vi "Read Children Tag.vi"(9 "Tag In":string, 11 "Tree in":refnum<class "Tree.lvclass">) -> (1 "Children Tag Out":string[](array[string]), 3 "Tree out":refnum<class "Tree.lvclass">)   [LabVIEW 2019, in "Tree.lvclass"]
uses:
  Tree.lvclass
  Tree.lvclass/Tree.ctl
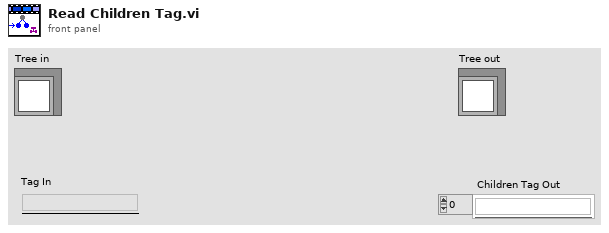
[diagram p1: front panel]
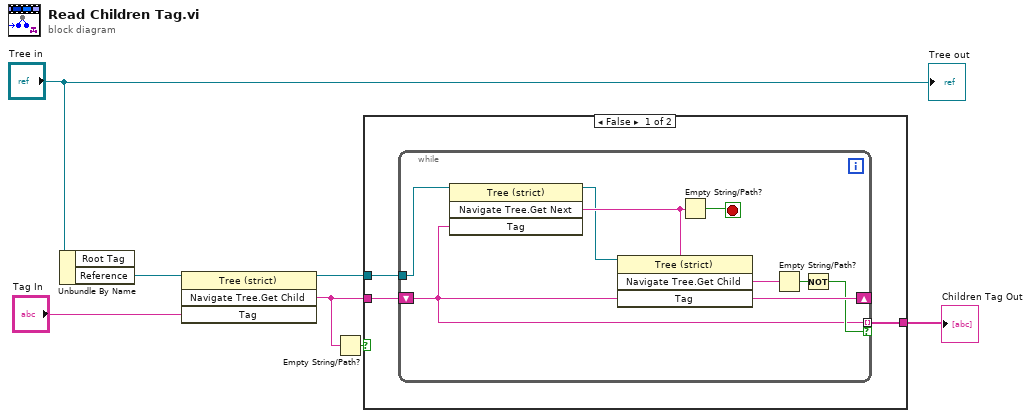
[diagram p0: block diagram]
diagram:
  n1 = Unbundle By Name("Tree in") -> ("Reference"=w7:refnum<vi>)  [unwired: 1 out]
  n2 = invoke class="Tree (strict)" method="Navigate Tree.Get Child"(reference=w7, "Tag"="Tag In") -> (reference out=w6:refnum<vi>, "Navigate Tree:Get Child"=w4:string)  [unwired: 2 in, 2 out]
  n3 = Empty String/Path?(string/path=w4) -> (empty?=w5:bool)
  n4 = case shown="False" w5 {
    tunnel: w4 -> [w10 _]
    tunnel: w6 -> [w9 _]
    tunnel: [w8 _] -> w2
    frame False {
      n5 = while {
        tunnel: w9 -> [w11]
        shift-right: [w18] -> _
        shift-left: w10 -> [w12]
        tunnel: [w12] -> w8 mode=indexing if=w13
        stop <- w17 stop-if-true
        n6 = invoke class="Tree (strict)" method="Navigate Tree.Get Next"(reference=w11, "Tag"=w12) -> (reference out=w16:refnum<vi>, "Navigate Tree:Get Next Item"=w18:string)  [unwired: 2 in, 2 out]
        n7 = invoke class="Tree (strict)" method="Navigate Tree.Get Child"(reference=w16, "Tag"=w12) -> ("Navigate Tree:Get Child"=w15:string)  [unwired: 2 in, 3 out]
        n8 = Empty String/Path?(string/path=w18) -> (empty?=w17:bool)
        n9 = Empty String/Path?(string/path=w15) -> (empty?=w14:bool)
        n10 = Not(x=w14) -> (.not. x?=w13:bool)
      }
    }
    frame True {
    }
  }
  "Children Tag Out" <- w2
  "Tree out" <- "Tree in"
